vi "calc_motors_shg.vi"(5 "fcu1_motor, f(x)":string, 7 "resonator_motor, f(x)":string="-2.10126553E+01 * x^2  + 6.31242686E+03 * x + 6.95582109E+05", 8 "error in (no error)":errorcluster, 10 "wavelength (nm)":dbl=355.0 format="%0.2f") -> (0 "error out":errorcluster, 1 "fcu1":i32, 2 "resonator":i32=288374)   [LabVIEW 2017, in "sirah.lvlib"]
uses:
  sirah.lvlib
  <vilib>/gmath/NI_Gmath.lvlib
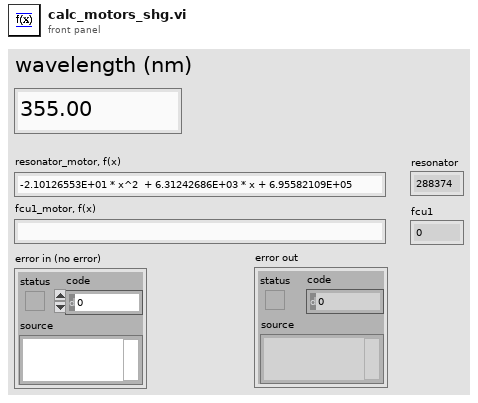
[diagram p1: front panel]
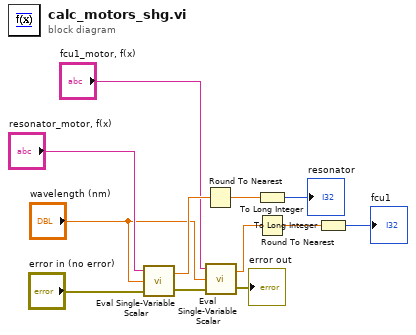
[diagram p0: block diagram]
diagram:
  n1 = call <vilib>:"Eval Single-Variable Scalar.vi"("error in (no error)"="error in (no error)", "x value"="wavelength (nm)", "formula"="resonator_motor, f(x)") -> ("error out"=w7:errorcluster, "y value"=w11:dbl)
  n2 = Round To Nearest(number=w11) -> (nearest integer value=w10:dbl)
  n3 = call <vilib>:"Eval Single-Variable Scalar.vi"("error in (no error)"=w7, "x value"="wavelength (nm)", "formula"="fcu1_motor, f(x)") -> ("error out"=→"error out":errorcluster, "y value"=w3:dbl)
  n4 = To Long Integer(number=w10) -> (32bit integer=→"resonator":i32)
  n5 = Round To Nearest(number=w3) -> (nearest integer value=w5:dbl)
  n6 = To Long Integer(number=w5) -> (32bit integer=→"fcu1":i32)
